vi "Display Timeout One Button Popup (SVG).vi"(4 "Message Size":T1={"Message Height"=-1, "Message Width"=-1, "Message Location"=enum."Bottom"} {"Message Width" min=-1 step=1; "Message Height" min=-1 step=1}, 6 "Theme":refnum<class "Theme.lvclass">, 7 "Button Text":string="OK", 8 "Error In":errorcluster, 9 "Timeout (s)":dbl=1.0, 10 "Message":string, 11 "Graphic":path) -> (0 "Error Out":errorcluster, 2 "Timeout":bool)   [LabVIEW 2021, in "Pop-Up.lvlib" / "SVG - Timeout One Button.lvclass"]
doc: "The custom timeout one button popup will display information to the user and wait for the operator to click the button or until the timeout expires.\n\n<b>Note:</b> This popup type allows the user to define a custom image for the display. The developer should test all settings prior to deployment to make sure that all images and text fit on the screen correctly.\n\n<b>Note:</b> The function <b>Close Pop-Up.vi</b> can be used to close this dialog early.\n\nInputs:\n-Graphic [path] - path to the image file to display\n-Message [String] - String Variable to populate Display with\n-Theme [lvclass] - the theme for the style of the popup\n-Message Info [typedef enum]\n -Message Height [I32] - the height for the message text box (-1 = match height of image)\n -Message Width [I32] - the width for the message text box (-1 = match height of image)\n -Message Location [Ring] - the location of the image relative to the message text box (left,\n right,bottom, top)\n-Button Text [string] - the text for the button\n-Timeout (s) [DBL] - timeout duration\n\n<b>Code Developed By:</b>\nDaniel Coons\nTechnology Service Corporation\n1983 S Liberty Drive\nBloomington, IN 47403\nPhone: 812 558-7100\ndaniel.coons@tsc.com\nwww.tsc.com/atcs"
uses:
  SVG - Timeout One Button.lvclass
  Theme/Theme.lvclass
  Popup/message info--typedef.ctl
  SVG - Timeout One Button.lvclass/SVG - Timeout One Button.ctl
  Popup/Popup.lvclass
  C:/Development/TSC.Pop-Up/SVG/SVG Parent.lvclass
  C:/Development/TSC.Pop-Up/Popup/Popup.lvclass
  C:/Development/TSC.Pop-Up/SVG/Custom/SVG - Timeout One Button/SVG - Timeout One Button.lvclass
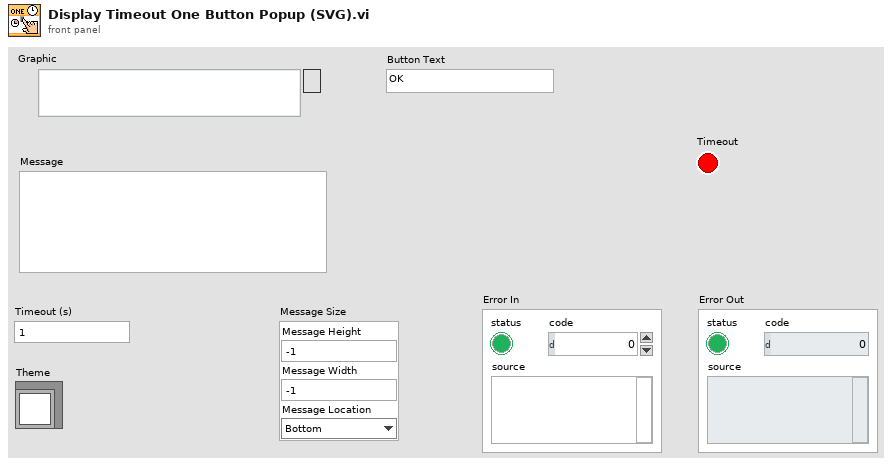
[diagram p1: front panel]
types:
  T1 = typedef "Pop-Up.lvlib/Popup.lvclass/message info--typedef.ctl" = cluster{"Message Height":i32, "Message Width":i32, "Message Location":enum16{"Top", "Bottom", "Right", "Left"}}
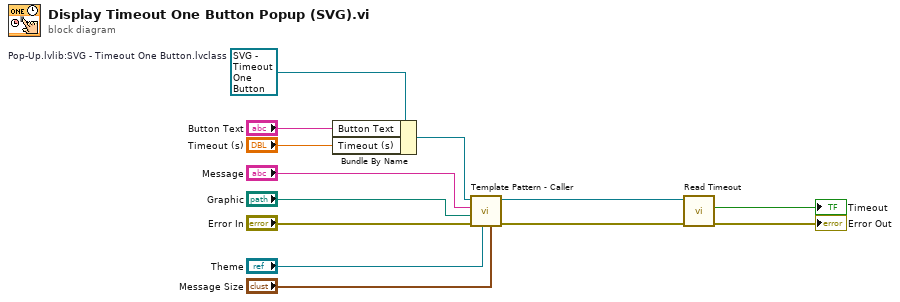
[diagram p0: block diagram]
diagram:
  w7 = refnum<class "SVG - Timeout One Button.lvclass"> refnum  # Pop-Up.lvlib:SVG - Timeout One Button.lvclass
  n1 = Bundle By Name(cluster=w7, "Button Text"="Button Text", "Timeout (s)"="Timeout (s)") -> (w8:refnum<class "SVG - Timeout One Button.lvclass">)
  n2 = call-dynamic "Template Pattern - Caller.vi"("Message Size"="Message Size", "Theme"="Theme", "error in (no error)"="Error In", "Graphic"="Graphic", "Message"="Message", "Pop-Up in"=w8) -> ("error out"=w9:errorcluster, "Pop-Up out"=w2:refnum<class "SVG - Timeout One Button.lvclass">)  [unwired: 4 in]
  n3 = call "Read Timeout.vi"("error in (no error)"=w9, "Popup in"=w2) -> ("error out"=→"Error Out":errorcluster, "Timeout?"=→"Timeout":bool)  [unwired: 7 in, 1 out]
